vi "validate key value pair.vi"(8 "error in":errorcluster, 9 "value":string, 10 "key":string, 11 "MotionModule configuration in":refnum<class "MotionModule configuration.lvclass">) -> (0 "error out":errorcluster, 3 "MotionModule configuration out":refnum<class "MotionModule configuration.lvclass">)   [LabVIEW 2017, in "MotionModule configuration.lvclass"]
uses:
  MotionModule configuration.lvclass
  <vilib>/NI/DCAF/Tag Editor Core/control module/configuration/control module configuration.lvclass
  Utilities/ProjectUtilities.lvlib
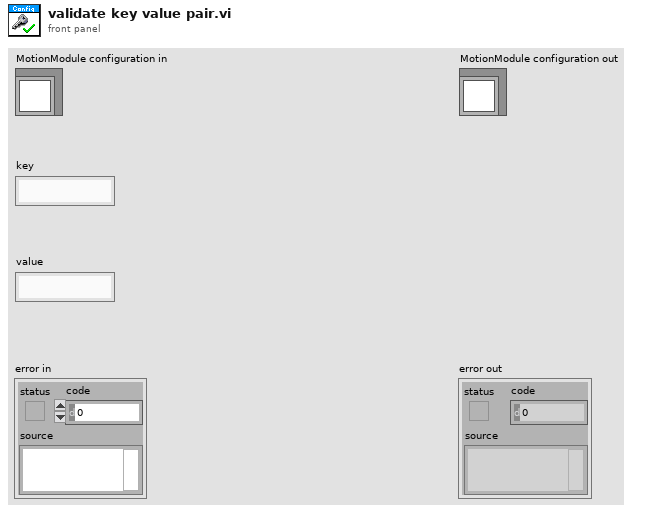
[diagram p1: front panel]
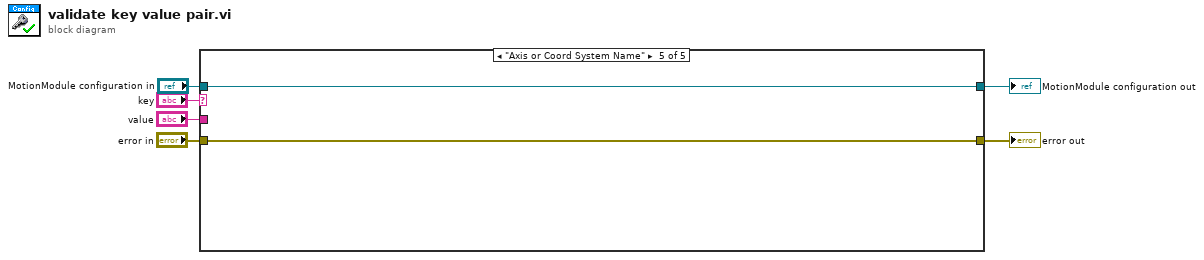
[diagram p0: block diagram]
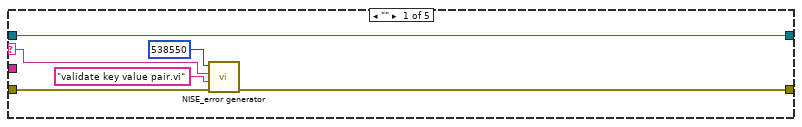
[diagram p2: hidden frame]
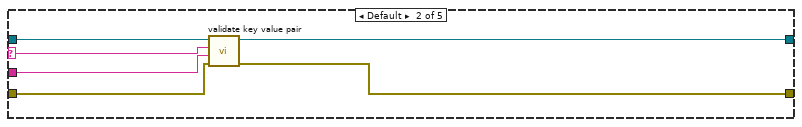
[diagram p3: hidden frame]
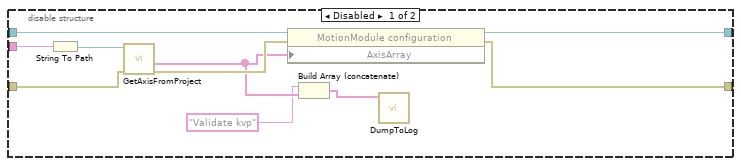
[diagram p5: hidden frame]
diagram:
  n1 = case shown="\"Axis or Coord System Name\"" "key" {
    selector: "key" -> [w9 w13 _ _ _]
    tunnel: [w7 w18 w20 w36 w38] -> w1
    tunnel: [w12 w17 w21 w37 w39] -> w6
    tunnel: "error in" -> [w8 w16 w22 w36 w38]
    tunnel: "value" -> [_ w15 w19 _ _]
    tunnel: "MotionModule configuration in" -> [w12 w14 w23 w37 w39]
    frame "" {
      n2 = call <vilib>:"NISE_error generator.vi"("error in"=w8, "source"="validate key value pair.vi", "append error message"=w9, "error code (0)"=538550) -> ("error out"=w7:errorcluster)  [unwired: 5 in]
    }
    frame Default {
      n3 = call-parent "validate key value pair.vi"("error in"=w16, "value"=w15, "key"=w13, "fixed channel configuration in"=w14) -> ("error out"=w18:errorcluster, "fixed channel configuration out"=w17:refnum<class "MotionModule configuration.lvclass">)  [unwired: 6 in]
    }
    frame "Path" {
      n4 = disable-structure shown="Enabled" {
        disable-tunnel: w23 -> [w33 w35]
        disable-tunnel: w22 -> [w31 w34]
        disable-tunnel: [w30 w35] -> w21
        disable-tunnel: [w28 w34] -> w20
        disable-tunnel: w19 -> [w24 _]
        frame Disabled {
          n5 = String To Path(string=w24) -> (path=w32:path)
          n6 = call "GetAxisFromProject.vi"("error in (no error)"=w31, "Path"=w32) -> ("error out"=w29:errorcluster, "Axis Array"=w27:string[])  [unwired: 7 in, 1 out]
          n7 = property class="MotionModule configuration"(reference=w33, error in=w29, "AxisArray"=w27) -> (reference out=w30:refnum<class "MotionModule configuration.lvclass">, error out=w28:errorcluster)
          n8 = Build Array (concatenate)("Validate kvp", w27) -> (w25:string[])
          n9 = call "DumpToLog.vi"("DataToLog"=w25) -> ()  [unwired: 11 in]
        }
        frame Enabled {
          # "#Dev: Disabling feature to get info from project."
        }
      }
    }
    frame "Axis In Coordinate System" {
    }
    frame "Axis or Coord System Name" {
    }
  }
  "error out" <- w1
  "MotionModule configuration out" <- w6
